vi "niRFUtil MASMT Util Get 2D CSG Type.vi"(1 "2D CSG Array in":csg[][](array[numeric])) -> (0 "2D CSG Array out":csg[][](array[numeric]))   [LabVIEW 2015, in "niRFUtil.lvlib"]
uses:
  niRFUtil.lvlib
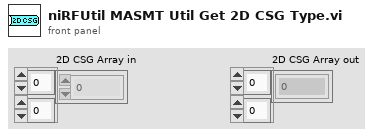
[diagram p1: front panel]
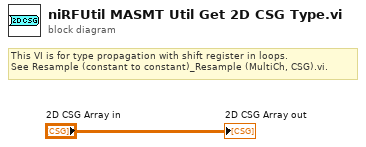
[diagram p0: block diagram]
diagram:
  # "This VI is for type propagation with shift register in loops.\nSee Resample (constant to constant)_Resample (MultiCh, CSG).vi."
  "2D CSG Array out" <- "2D CSG Array in"
